vi "Analysis.Tab.vi"() -> ()   [LabVIEW 2015, in "Analysis.lvlib"]
uses:
  Analysis.lvlib
  Types/Analysis.GUI.Parameters.ctl
  Types/Analysis.StateVariables.ctl
  Types/Analysis.GUI.Refs.ctl
  <vilib>/NI/AMC/Read Termination Message.vi
  <vilib>/NI/AMC/Create Single Message.vi
  <vilib>/NI/AMC/Update Message Routing Info.vi
  <vilib>/NI/AMC/Create Multiple Messages.vi
  <vilib>/NI/AMC/Globals.vi
  <vilib>/NI/AMC/Send Message.vi
  <vilib>/NI/AMC/AMC.lvlib
panel:
  in  "Parameters":T1={"Results Path"=path "C:/testdata/Logs", "Temp Path"=path "C:/testdata/Temp", "Remote Path"=path "d:/testdata/Logs", "Analysis VIs"=[path "C:/addons/TestStand Examples for HIL/Continuous Monitoring Tester/Sequences/Analysis/Builds/TestStand Analysis Steps.lvlibp/Post Process Analysis Steps/Analysis.LevelTransition.vi"], "Report Passed?"=FALSE, "Group Channels?"=FALSE}
  out "Results Directory":path=path "d:/testdata/TestResults"
  out "Cycle":i32
  in  "Results":string(tree)
  out "Station ID":string="Station 1"
  in  "Station.ID":string="All"
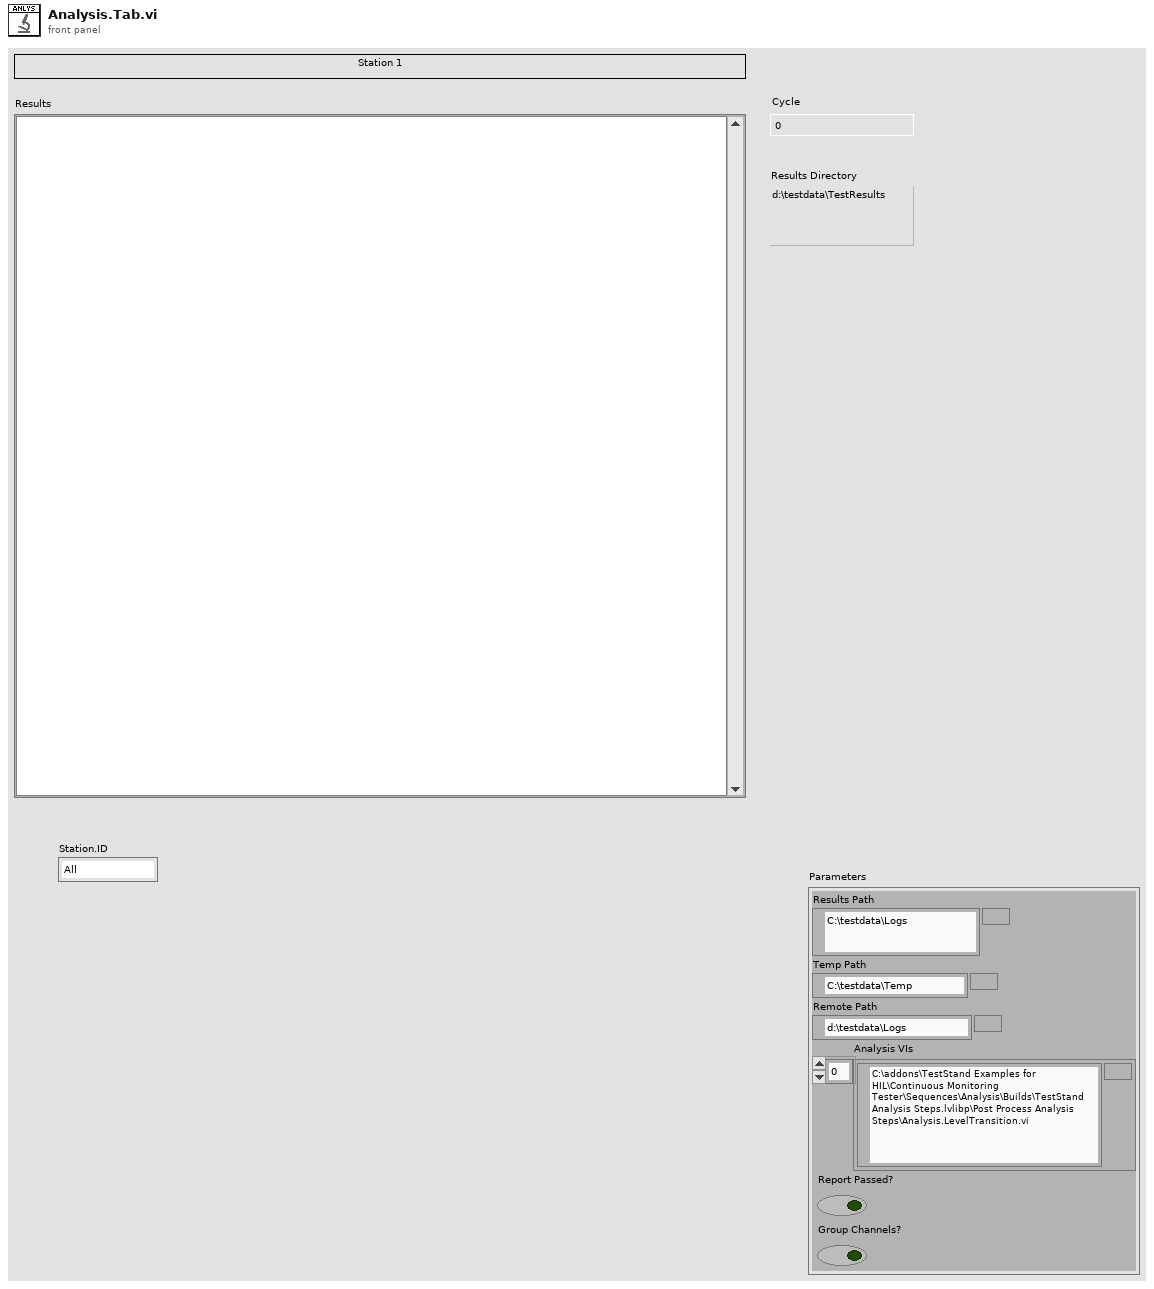
[diagram p1: front panel]
types:
  T1 = typedef "Analysis.lvlib/Analysis.GUI.Parameters.ctl" = cluster{"Results Path":path, "Temp Path":path, "Remote Path":path, "Analysis VIs":path[], "Report Passed?":bool, "Group Channels?":bool}
  T2 = typedef "Analysis.lvlib/Analysis.GUI.Refs.ctl" = cluster{"Cycle":refnum<vi>, "Tree":refnum<vi>, " VI":refnum<vi>, "Results.Directory":refnum<vi>}
  T3 = typedef "Analysis.lvlib/Analysis.StateVariables.ctl" = cluster{"Boolean":bool}
  T4 = typedef "AMC.lvlib/Message Queue.ctl" = refnum<queue>
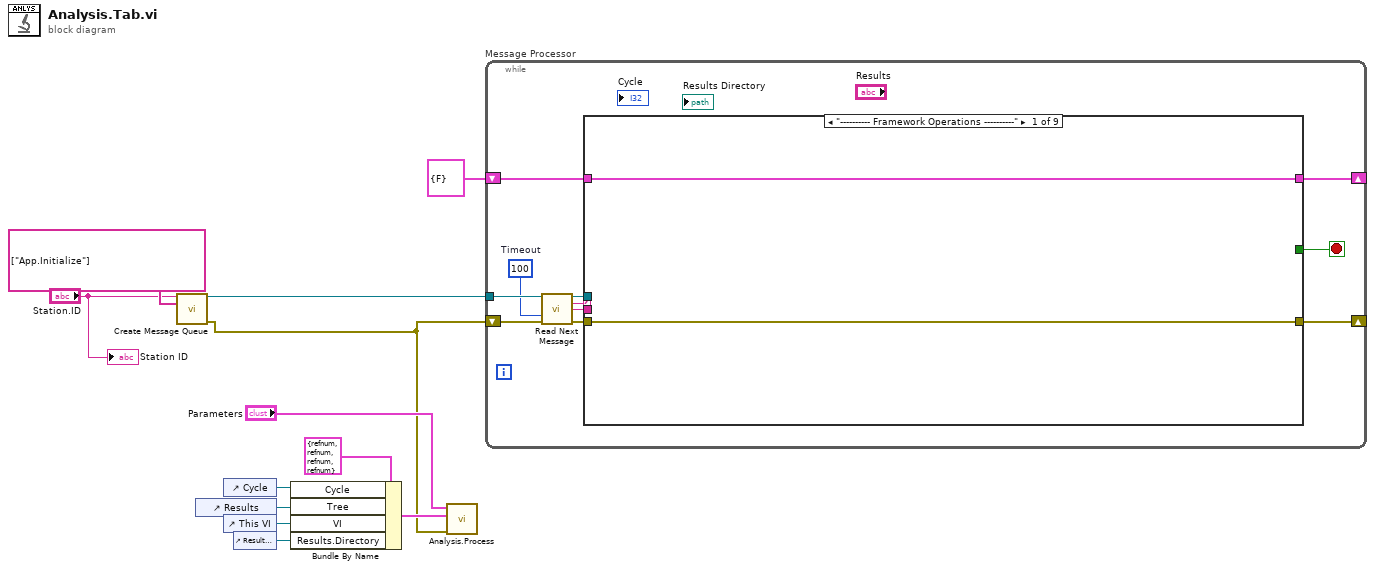
[diagram p0: block diagram]
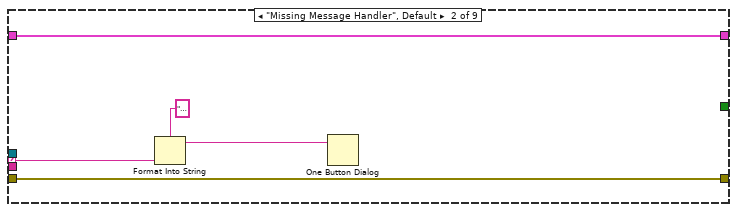
[diagram p2: hidden frame]
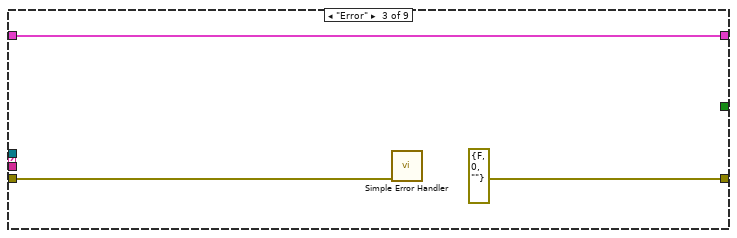
[diagram p3: hidden frame]
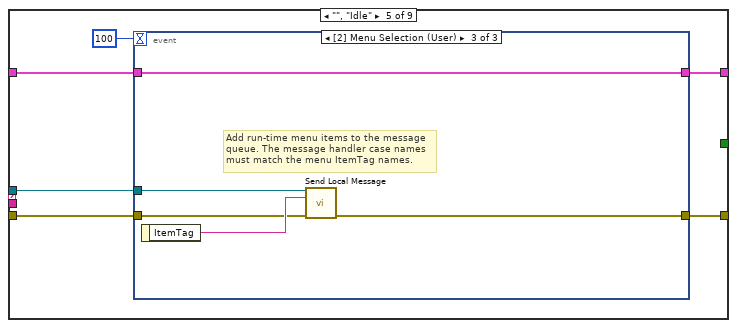
[diagram p5: hidden frame]
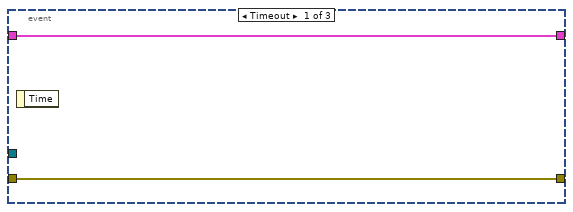
[diagram p6: hidden frame]
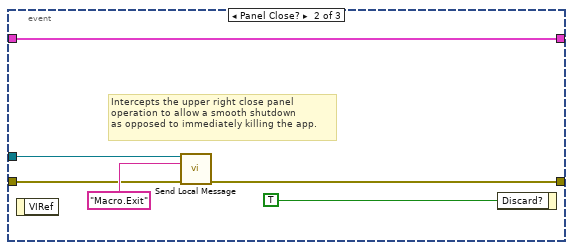
[diagram p7: hidden frame]
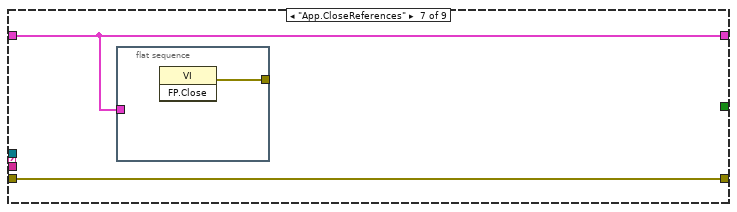
[diagram p9: hidden frame]
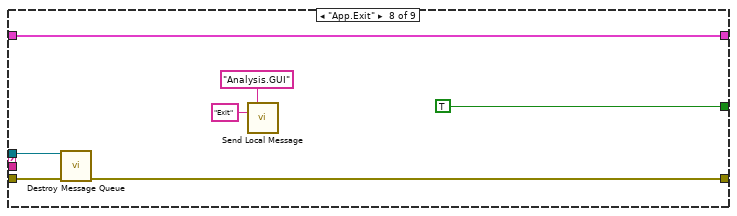
[diagram p10: hidden frame]
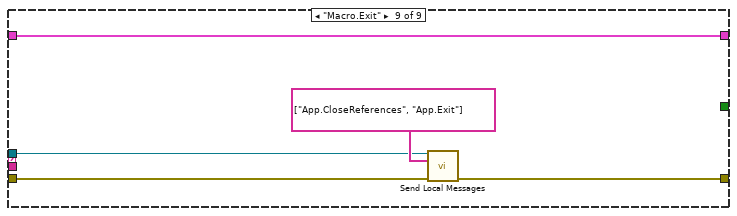
[diagram p11: hidden frame]
diagram:
  n1 = call <vilib>:"Create Message Queue.vi"("message queue name"="Station.ID", "initial message names"=string[] ["App.Initialize"]) -> ("message queue out"=w11:T4, "error out"=w2:errorcluster)  [unwired: 12 in]
  n2 = control-ref of="Results"() -> (w4:refnum<vi>)
  n3 = control-ref of="Cycle"() -> (w5:refnum<vi>)
  n4 = control-ref of="This VI"() -> (w8:refnum<vi>)
  n5 = control-ref of="Results Directory"() -> (w3:refnum<vi>)
  n6 = Bundle By Name(cluster=T2 {"Cycle"=refnum, "Tree"=refnum, " VI"=refnum, "Results.Directory"=refnum} ("output cluster"), "Cycle"=w5, "Tree"=w4, "VI"=w8, "Results.Directory"=w3) -> (w6:T2)
  n7 = call "Analysis.Process.vi"("error in (no error)"=w2, "Refs"=w6, "Parameters"="Parameters") -> ()  [unwired: 9 in]
  n8 = while "Message Processor" {
    shift-left: w2 -> [w18]
    shift-right: [w21] -> _
    tunnel: w11 -> [w19]
    shift-left: T3 {"Boolean"=FALSE} ("state variables") -> [w23]
    shift-right: [w22] -> _
    stop <- w13 stop-if-true
    w14 = 100  # Timeout
    n9 = call <vilib>:"Read Next Message.vi"("message queue in"=w19, "timeout (1 ms)"=w14, "error in"=w18) -> ("message queue out"=w20:T4, "message name"=w16:string, "message value"=w15:string, "error out"=w17:errorcluster)  [unwired: 5 in, 4 out]
    n10 = case shown="\"---------- Framework Operations ----------\"" w16 {
      selector: w16 -> [_ w28 _ _ _ _ _ _ _]
      tunnel: [w25 w30 w33 w35 w36 w55 w57 w66 w71] -> w22
      tunnel: w23 -> [w25 w30 w33 w35 w37 w55 w57 w66 w71]
      tunnel: w20 -> [_ _ _ _ w41 _ _ w64 w67]
      tunnel: w17 -> [w24 w29 w31 w34 w40 w56 w58 w65 w69]
      tunnel: [w24 w29 errorcluster {"status"=FALSE, "code"=0, "source"=""} ("error out") w34 w39 w56 w58 w63 w68] -> w21
      tunnel: w15 -> [_ _ _ _ _ _ _ _ _]
      tunnel: [_ _ _ _ _ _ _ TRUE _] -> w13
      frame "---------- Framework Operations ----------" {
      }
      frame "Missing Message Handler", Default {
        n11 = Format Into String(format string="DevError: Missing message handler for '%s\" message." ("message"), w28) -> (resulting string=w26:string)  [unwired: 2 in, 1 out]
        n12 = One Button Dialog(message=w26) -> ()  [unwired: 2 out]
      }
      frame "Error" {
        n13 = call <vilib>:"Simple Error Handler.vi"("error in (no error)"=w31) -> ()  [unwired: 1 in, 8 out]
      }
      frame "---------- Application Operations ----------" {
      }
      frame "", "Idle" {
        n14 = event shown="[2] Menu Selection (User)" {
          selector: _ -> [_ _ _]
          dyn-events: _ -> [_ _ _]
          timeout: 100 -> [_ _ _]
          tunnel: w41 -> [_ w47 w53]
          tunnel: w40 -> [w43 w46 w52]
          tunnel: [w43 w45 w51] -> w39
          tunnel: w37 -> [w42 w44 w50]
          tunnel: [w42 w44 w50] -> w36
          event Timeout {
            n15 = event-data() -> ()  [unwired: 2 out]
          }
          event Panel Close? {
            # "Intercepts the upper right close panel\noperation to allow a smooth shutdown\nas opposed to immediately killing the app."
            n16 = event-data() -> ()  [unwired: 2 out]
            n17 = call <vilib>:"Send Local Message.vi"("message queue in"=w47, "message name"="Macro.Exit", "error in"=w46) -> ("error out"=w45:errorcluster)  [unwired: 10 in, 2 out]
            n18 = event-data("Discard?"=TRUE) -> ()  [unwired: 1 in, 1 out]
          }
          event Menu Selection (User) {
            # "Add run-time menu items to the message\nqueue. The message handler case names must match the menu ItemTag names."
            n19 = event-data() -> ("ItemTag"=w54:string)  [unwired: 1 out]
            n20 = call <vilib>:"Send Local Message.vi"("message queue in"=w53, "message name"=w54, "error in"=w52) -> ("error out"=w51:errorcluster)  [unwired: 10 in, 2 out]
          }
        }
      }
      frame "App.Initialize" {
      }
      frame "App.CloseReferences" {
        n21 = flat-sequence {
          tunnel: w57 -> [_]
          tunnel: [w59] -> _
          frame #0 {
            n22 = invoke class="VI" method="FP.Close"() -> (error out=w59:errorcluster)  [unwired: 3 in, 2 out]
          }
        }
      }
      frame "App.Exit" {
        n23 = call <vilib>:"Destroy Message Queue.vi"("message queue in"=w64, "error in"=w65) -> ("error out"=w63:errorcluster)  [unwired: 11 in, 2 out]
        n24 = call <vilib>:"Send Local Message.vi"("receiver process (\"\" - local)"="Analysis.GUI" ("message queue name"), "message name"="Exit") -> ()  [unwired: 11 in, 3 out]
      }
      frame "Macro.Exit" {
        n25 = call <vilib>:"Send Local Messages.vi"("message queue in"=w67, "message names"=string[] ["App.CloseReferences", "App.Exit"], "error in"=w69) -> ("error out"=w68:errorcluster)  [unwired: 10 in, 2 out]
      }
    }
  }
  "Station ID" <- "Station.ID"
